vi "on.vi"(0 "reference in":refnum<class "active object queue.lvclass">, 5 "error in (no error)":errorcluster) -> (14 "reference out":refnum<class "active object queue.lvclass">, 19 "error out":errorcluster)   [LabVIEW 2019, in "active object queue.lvclass"]
uses:
  active object queue.lvclass
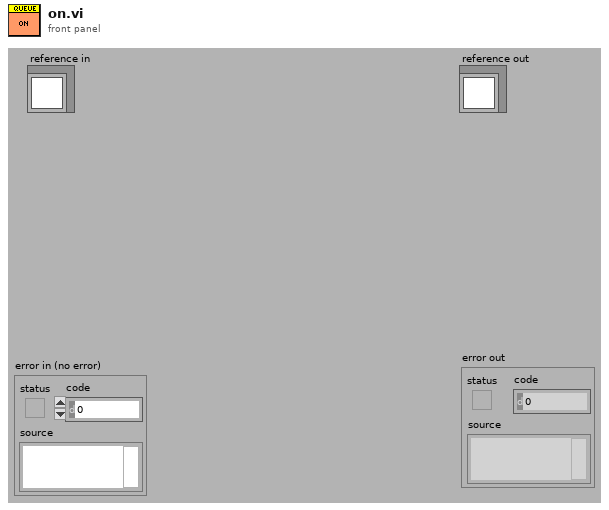
[diagram p1: front panel]
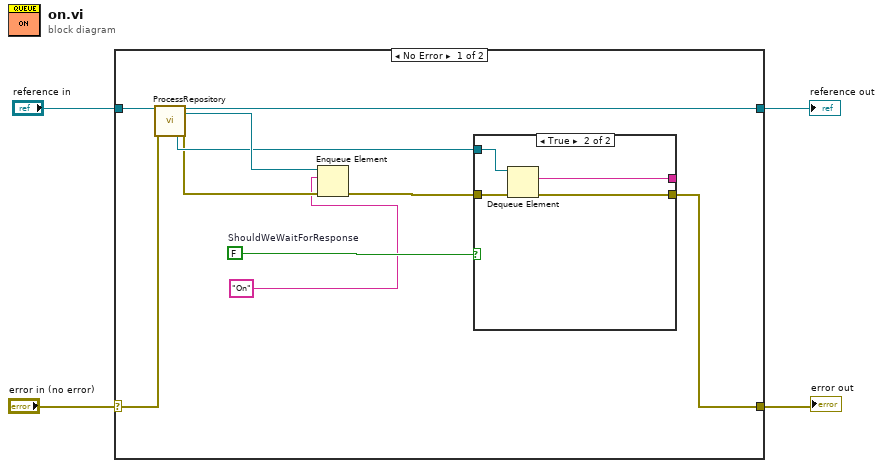
[diagram p0: block diagram]
diagram:
  n1 = case shown="No Error" "error in (no error)" {
    selector: "error in (no error)" -> [w14 w21]
    tunnel: [w6 w21] -> w3
    tunnel: [w12 w20] -> w1
    tunnel: "reference in" -> [w13 w20]
    frame No Error {
      w10 = FALSE  # ShouldWeWaitForResponse
      n2 = call "ProcessRepository.vi"("reference in"=w13, "error in (no error)"=w14) -> ("FromProcessQueue"=w8:refnum<queue>, "reference out"=w12:refnum<class "active object queue.lvclass">, "ToProcessQueue"=w11:refnum<queue>, "error out"=w7:errorcluster)  [unwired: 11 in, 3 out]
      n3 = Enqueue Element(queue=w11, element="On" ("MessageToProcess"), error in (no error)=w7) -> (error out=w9:errorcluster)  [unwired: 1 in, 2 out]
      n4 = case shown="True" w10 {
        tunnel: w9 -> [w15 w19]
        tunnel: w8 -> [_ w18]
        tunnel: [_ w17] -> _
        tunnel: [w15 w16] -> w6
        frame False {
        }
        frame True {
          n5 = Dequeue Element(queue=w18, error in (no error)=w19) -> (element=w17:string, error out=w16:errorcluster)  [unwired: 1 in, 2 out]
        }
      }
    }
    frame Error {
    }
  }
  "error out" <- w3
  "reference out" <- w1
